vi "LSX Get Limit.vi"(7 "pdMaxRange":dbl, 8 "error in (no error)":errorcluster, 9 "pdMinRange":dbl, 10 "lAxis":i32, 11 "lLSID":i32) -> (0 "error out":errorcluster, 1 "pdMinRange out":dbl, 3 "function return":i32, 5 "pdMaxRange out":dbl)   [LabVIEW 2018, in "Tango.lvlib"]
doc: "TANGOAPI int TANGOCALL LSX_GetLimit (int lLSID, int lAxis, double *pdMinRange, double *pdMaxRange);"
uses:
  Tango.lvlib
  SubVIs/Tango_DLL.dll
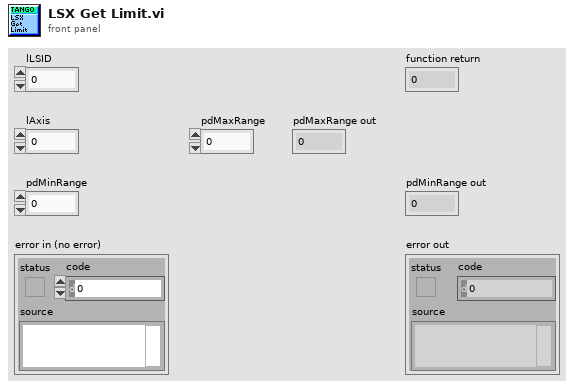
[diagram p1: front panel]
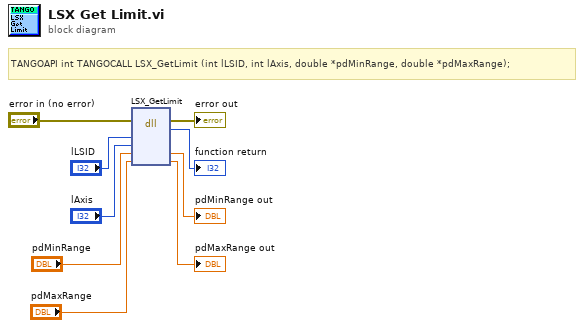
[diagram p0: block diagram]
diagram:
  # "TANGOAPI int TANGOCALL LSX_GetLimit (int lLSID, int lAxis, double *pdMinRange, double *pdMaxRange);"
  n1 = dll-call lib="C:/Users/Familie/Documents/LabviewIX81/lib/TANGO Stage/SubVIs/Tango_DLL.*" fn="LSX_GetLimit"(error in="error in (no error)", "lLSID"="lLSID", "lAxis"="lAxis", "pdMinRange"="pdMinRange", "pdMaxRange"="pdMaxRange") -> (error out=→"error out":errorcluster, →"function return":i32, "pdMinRange"=→"pdMinRange out":dbl, "pdMaxRange"=→"pdMaxRange out":dbl)  [unwired: 4 in, 1 out]
